vi "CCE T022 SubVI01.vi"(11 "Tensión":dbl(slide) scale=-12.0..12.0) -> (3 "Posicion":dbl(knob))   [LabVIEW 2020]
doc: "Ceballos Conde Emanuel 4MV6 Sistemas de visión artificial 2022/1\nEste VI contiene el modelo de un motor de corriente directa"
panel:
  in  "y":dbl=10.0 format="%#_13g"
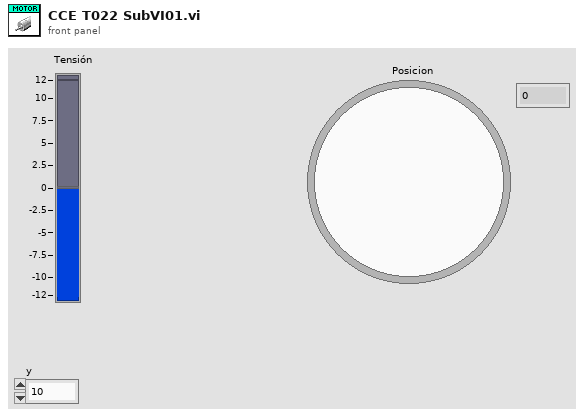
[diagram p1: front panel]
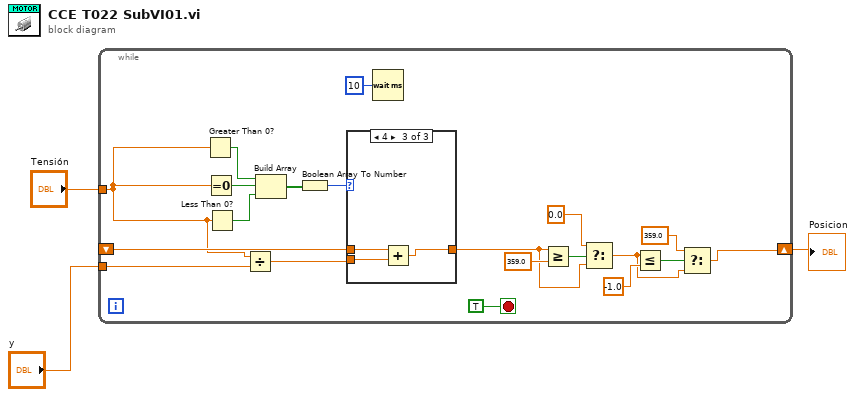
[diagram p0: block diagram]
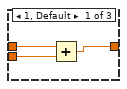
[diagram p2: hidden frame]
diagram:
  n1 = while {
    shift-right: [w8] -> w2
    shift-left: _ -> [w17]
    tunnel: "Tensión" -> [w5]
    tunnel: "y" -> [w4]
    stop <- TRUE stop-if-true
    n2 = Greater Than 0?(x=w5) -> (x > 0?=w21:bool)
    n3 = Equal To 0?(x=w5) -> (x = 0?=w22:bool)
    n4 = Less Than 0?(x=w5) -> (x < 0?=w20:bool)
    n5 = Divide(x=w5, y=w4) -> (x/y=w7:dbl)
    n6 = Build Array(w21, w22, w20) -> (w19:bool[])
    n7 = Boolean Array To Number(Boolean array=w19) -> (number=w18:u32)
    n8 = case shown="4" w18 {
      tunnel: w17 -> [w26 w27 w30]
      tunnel: [w24 w27 w28] -> w13
      tunnel: w7 -> [w25 _ w29]
      frame 1, Default {
        n9 = Add(x=w26, y=w25) -> (x+y=w24:dbl)
      }
      frame 2 {
      }
      frame 4 {
        n10 = Add(x=w30, y=w29) -> (x+y=w28:dbl)
      }
    }
    n11 = Wait (ms)(milliseconds to wait=u32 10) -> ()  [unwired: 1 out]
    n12 = Greater Or Equal?(x=w13, y=359.0) -> (x >= y?=w15:bool)
    n13 = Select(t=0.0, s=w15, f=w13) -> (s? t:f=w9:dbl)
    n14 = Less Or Equal?(x=w9, y=-1.0) -> (x <= y?=w11:bool)
    n15 = Select(t=359.0, s=w11, f=w9) -> (s? t:f=w8:dbl)
  }
  "Posicion" <- w2
